vi "servo_park_squence.vi"(0 "servo 3":u8) -> ()   [LabVIEW 2017]
uses:
  GlobalVar.vi
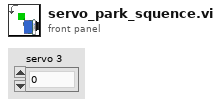
[diagram p1: front panel]
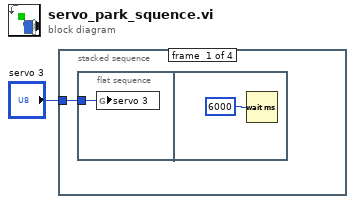
[diagram p0: block diagram]
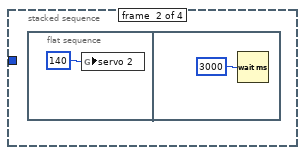
[diagram p2: hidden frame]
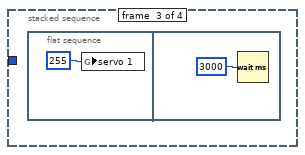
[diagram p3: hidden frame]
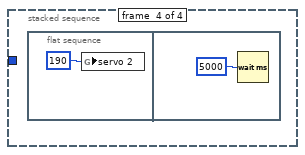
[diagram p4: hidden frame]
diagram:
  n1 = stacked-sequence {
    tunnel: "servo 3" -> [w2 _ _ _]
    frame #0 {
      n2 = flat-sequence {
        tunnel: w2 -> [w3]
        frame #0 {
          n3 = global write "GlobalVar.vi" "servo 3"(w3) -> ()
        }
        frame #1 {
          n4 = Wait (ms)(milliseconds to wait=u32 6000) -> ()  [unwired: 1 out]
        }
      }
    }
    frame #1 {
      n5 = flat-sequence {
        frame #0 {
          n6 = global write "GlobalVar.vi" "servo 2"(u8 140 ("servo 1")) -> ()
        }
        frame #1 {
          n7 = Wait (ms)(milliseconds to wait=u32 3000) -> ()  [unwired: 1 out]
        }
      }
    }
    frame #2 {
      n8 = flat-sequence {
        frame #0 {
          n9 = global write "GlobalVar.vi" "servo 1"(u8 255 ("servo 1")) -> ()
        }
        frame #1 {
          n10 = Wait (ms)(milliseconds to wait=u32 3000) -> ()  [unwired: 1 out]
        }
      }
    }
    frame #3 {
      n11 = flat-sequence {
        frame #0 {
          n12 = global write "GlobalVar.vi" "servo 2"(u8 190 ("servo 1")) -> ()
        }
        frame #1 {
          n13 = Wait (ms)(milliseconds to wait=u32 5000) -> ()  [unwired: 1 out]
        }
      }
    }
  }
